vi "BeamCal.vi"() -> ()   [LabVIEW 2022 SP3]
uses:
  -CalTransducer/Hydros.ctl
  -CalTransducer/HydrophoneSettings.ctl
  <vilib>/Analysis/baseanly.llb/Mean (DBL).vi
  <vilib>/Utility/file.llb/Write Delimited Spreadsheet (DBL).vi
  <vilib>/Analysis/2dsp.llb/Zero Padder (DBL).vi
  <vilib>/Analysis/NI_AALPro.lvlib
  <vilib>/Analysis/NI_AALBase.lvlib
panel:
  in  "x*y":dbl[](array[numeric])
  in  "Save P profile":bool
  out "+- Pres":dbl[][](graph)
  in  "Save Path":path
  in  "Next File":bool
  in  "Save Time":bool
  in  "Save Spectra":bool
  in  "View Header?":bool
  in  "Pulse Thresh":dbl=0.025
  out "Data Summary":dbl[](array[numeric])
  in  "ExitSendCmd":bool
  in  "Scale Src":u16(ring)=2 items=["Enter Peak Voltage", "Pk from RF Att ", "Pk from Volt pram"]
  in  "booster amp?":bool=TRUE
  out "Power Spectrum":T1(graph)
  out "StopFreq":dbl format="%.2f"
  out "StartFreq":dbl format="%.2f"
  out "Bandwidth (MHz)\n(6 dB)":dbl format="%.2f"
  out "Max Pulse Parameters":T2 {"pos peak pressure (MPa)" format="%.2f"; "focal length (cm)" format="%.2f"; "MI" format="%.2f"; "Ita.3" format="%.2f"; "Temporal Av Intensity \n(Ita mW/cm^2)" format="%.2f"; "Ipa.3" format="%.2f"; "Pulse Av Intensity\n (Ipa W/cm^2)" format="%.2f"; "Pulse Int \nIntegral (PII J/cm^2)" format="%.2e"; "pulse dur (Pd s)" format="%.3e"; "p.3" format="%.2f"; "neg peak pressure (MPa)" format="%.3f"; "derating (.3) factor" format="%.2f"; "prf" format="%.2f"; "Frequency (MHz)" format="%.2f"}
  out "Power (mW)":dbl format="%.2e"
  in  "Save to file":bool
  out "Isata (mW/cm^2)":dbl format="%.2f"
  in  "pk votage scale (V)":dbl=0.2 format="%.3f"
  out "Raw data":dbl[][](graph)
  out "max line":i32=64
  in  "Hydrophone":T3=enum."DEAD PAL #1818"
  out "beamwidth micron\n(6 dB)":dbl format="%.2f"
  out "Ita":dbl[](graph)
  in  "prf":dbl=1000.0 format="%.2f"
  out "window duration (s)":dbl format="%.2e"
  out "Line":dbl[](graph)
  in  "new file path":path
  in  "Cal Freq (MHz)":dbl=1.0 format="%.2f"
  # "Data is normalized to value of negative peak pressure"
  # "1. Open File (click file image for new path).\n2. Enter parameters (colored fields).\n3. Set Yellow and Red cursors to span pulse.\n4. Adjust Pulse Thresh if necessary.\n5. Most inputs are dynamic and will change values.\n6. To save data, select Save to File on and run VI."
  # "***Voltages are inverted for 40 um PAL devices***"
  # "beam cross sectional\npower"
  # "© 2000-2017 WCM"
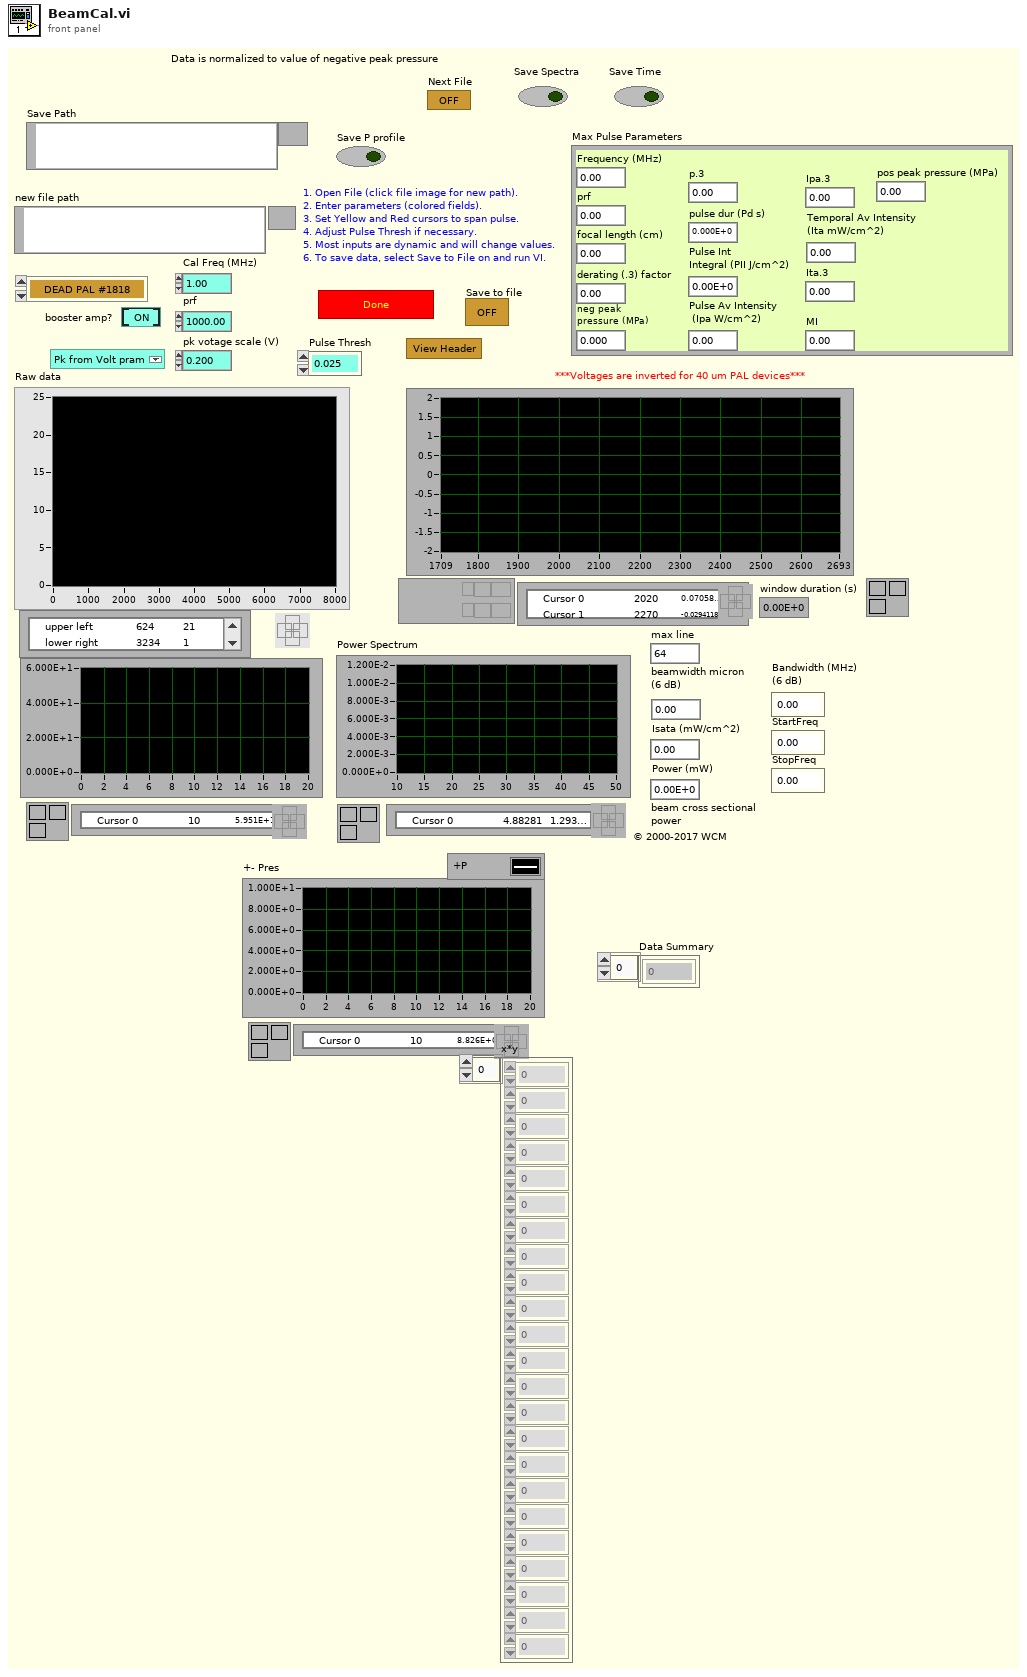
[diagram p1: front panel]
types:
  T1 = cluster{i32, "df":dbl, "Power Spectrum (V^2 rms)":dbl[]}
  T2 = cluster{"Frequency (MHz)":dbl, "prf":dbl, "focal length (cm)":dbl, "derating (.3) factor":dbl, "neg peak pressure (MPa)":dbl, "pos peak pressure (MPa)":dbl, "p.3":dbl, "pulse dur (Pd s)":dbl, "Pulse Int \nIntegral (PII J/cm^2)":dbl, "Pulse Av Intensity\n (Ipa W/cm^2)":dbl, "Ipa.3":dbl, "Temporal Av Intensity \n(Ita mW/cm^2)":dbl, "Ita.3":dbl, "MI":dbl}
  T3 = typedef "Hydros.ctl" = enum16{"PAL #1048", "PAL #525", "PAL #430a", "PAL #192", "DEAD PAL # 1403", "LOST UHI Onda", "DEAD PAL #1818", "PAL #1974", "DEAD #2266 w/booster", "PAL #2524 w/booster", "PAL FP21-20T", "PAL FP160-13  ", "PAL FP141-20", "PAL FP158-08T"}
  T4 = typedef "HydrophoneSettings.ctl" = cluster{"Center Freq (MHz)":dbl, "PRF (kHz)":dbl, "Pulse window (us)":dbl, "Hydrophone":T3, "booster amp?":bool}
  T5 = enum16{"open", "open or create", "create or replace", "create", "open (read only)"}
  T6 = typedef "Header.ctl" = cluster{"header info":cluster{"Header":string, "Head length":i16}, "A/D info":cluster{"# rf points per line":u16, "# lines per scan":u16, "sample rate MHz":u16, "# A/D bits":i16, "# bytes per A/D":u16, "TGC Flag":u16, "A/D Type":string}, "Tranducer Info":cluster{"bandwidth":sgl, "center freq":sgl, "start freq":sgl, "ID":i32}, "Scan Info":cluster{"delay":sgl, "pivot distance":sgl, "sector scan angle":sgl, "operator":string, "Scan Mode":string, "location":string}, "Time/Date Info":cluster{"date":string, "time":string}, "RF Info":cluster{"RF file name":string, "RF file att":string, "RF cal file name":string, "RF cal file att":string}, "Patient Info":cluster{"ID":string, "extended ID":string, "age":u16, "sex":string, "previously\nscanned":string, "PSA":sgl, "LOS":u8, "Ethnicty 2":u8, "Race":u8}, "Tissue Type":cluster{"organ":i16, "disease type":i16, "disease location":i16, "IQ_pts":u16, "RcvBuffer":u8, "RcvFrame":u16, "IQBuff":u8, "IQFrame":u16, "IQPage":u8}, "Votage scaling":cluster{"Digitizer (dB)":sgl, "Gain (dB)":sgl, "Atten (dB)":sgl}, "Comment":string, "Misc Info":cluster{"avg num":u16, "c speed":i16, "Div By or SF zones":i16, "XMIT CHS":u8, "RCV CHS":u8, "Xmit angle":sgl}, "Therapy Parameters":cluster{"Theraputic Freq (MHz)":sgl, "Time on (s)":sgl, "Therapy amplitude (mV)":sgl, "Lines Before":u16, "Lines After":u16}, "Scan Settings":cluster{"Energy (uJ or V)":u8, "Damp (Ohm) or Fc":u8, "HP Filt (KHz)":u8, "LP Filt (MHz)":u8, "Gain (db)":u8, "prf (kHz)":sgl, "Distance between\nscan lines (um)":u16, "Distance between\nscan planes (um)":u16, "Scan line gap (um)":sgl, "Scan plane gap (um)":sgl}, "Compression Parameters":cluster{"F1 (MHz)":sgl, "F2 (MHz)":sgl, "% taper":sgl, "duration":sgl}, "Patient Info Xtra":cluster{"First Name":string, "Last Name":string, "Notes":string}, "ROI Box":u16[]}
  T7 = typedef "LVCursorListTypeDef.ctl" = cluster{"Name":string, "Color":u32, "Style":u8, "Point Style":u8, "Name Visible":bool, "Allow Drag":bool, "Cursor Mode":u32, "Plot":i32, "Index":i32, "Position":cluster{"X":dbl, "Y":dbl}, "X Scale":u32, "Y Scale":u32, "Watch Plots":i32[], "Watch All Plots":bool, "Plot Area":i32, "Label Offset":cluster{"X":dbl, "Y":dbl}}[]
  T8 = cluster{"Name":string, "Color":u32, "Style":u8, "Point Style":u8, "Name Visible":bool, "Allow Drag":bool, "Cursor Mode":u32, "Plot":i32, "Index":i32, "Position":cluster{"X":dbl, "Y":dbl}, "X Scale":u32, "Y Scale":u32, "Watch Plots":i32[], "Watch All Plots":bool, "Plot Area":i32, "Label Offset":cluster{"X":dbl, "Y":dbl}}
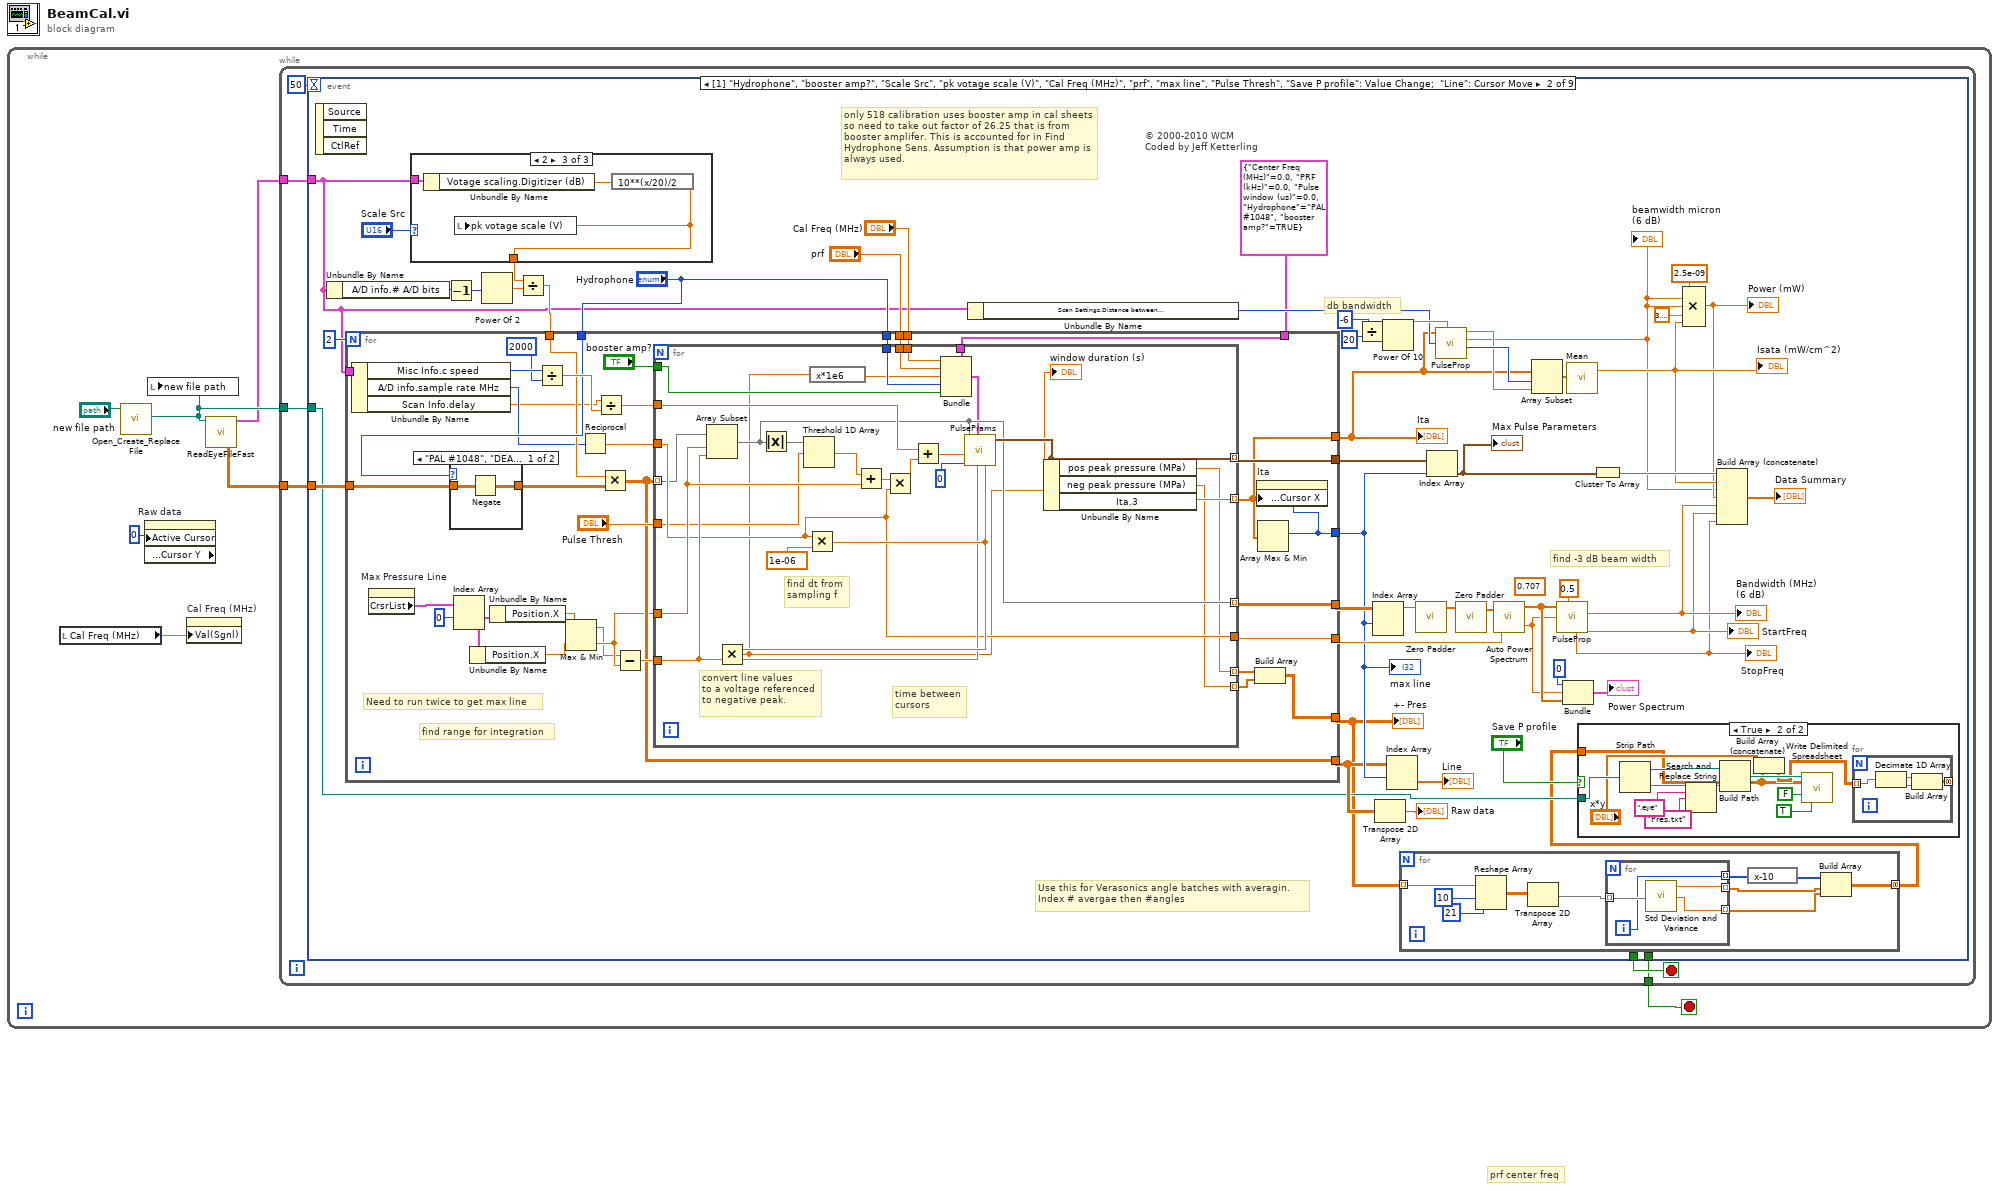
[diagram p0: block diagram]
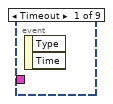
[diagram p2: hidden frame]
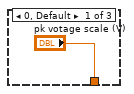
[diagram p5: hidden frame]
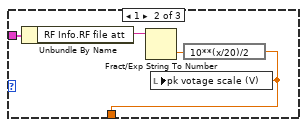
[diagram p6: hidden frame]
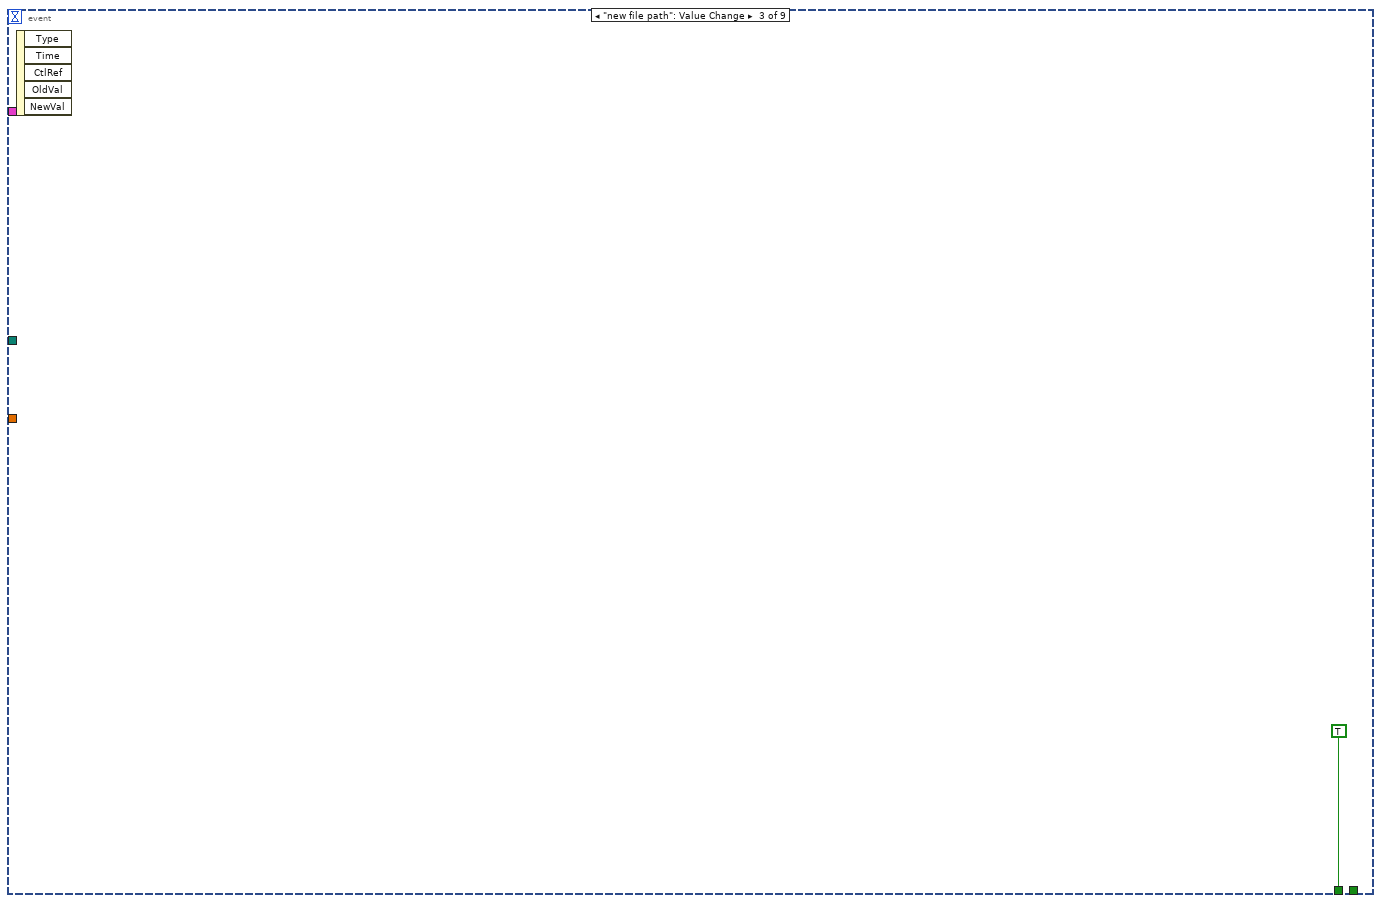
[diagram p7: hidden frame]
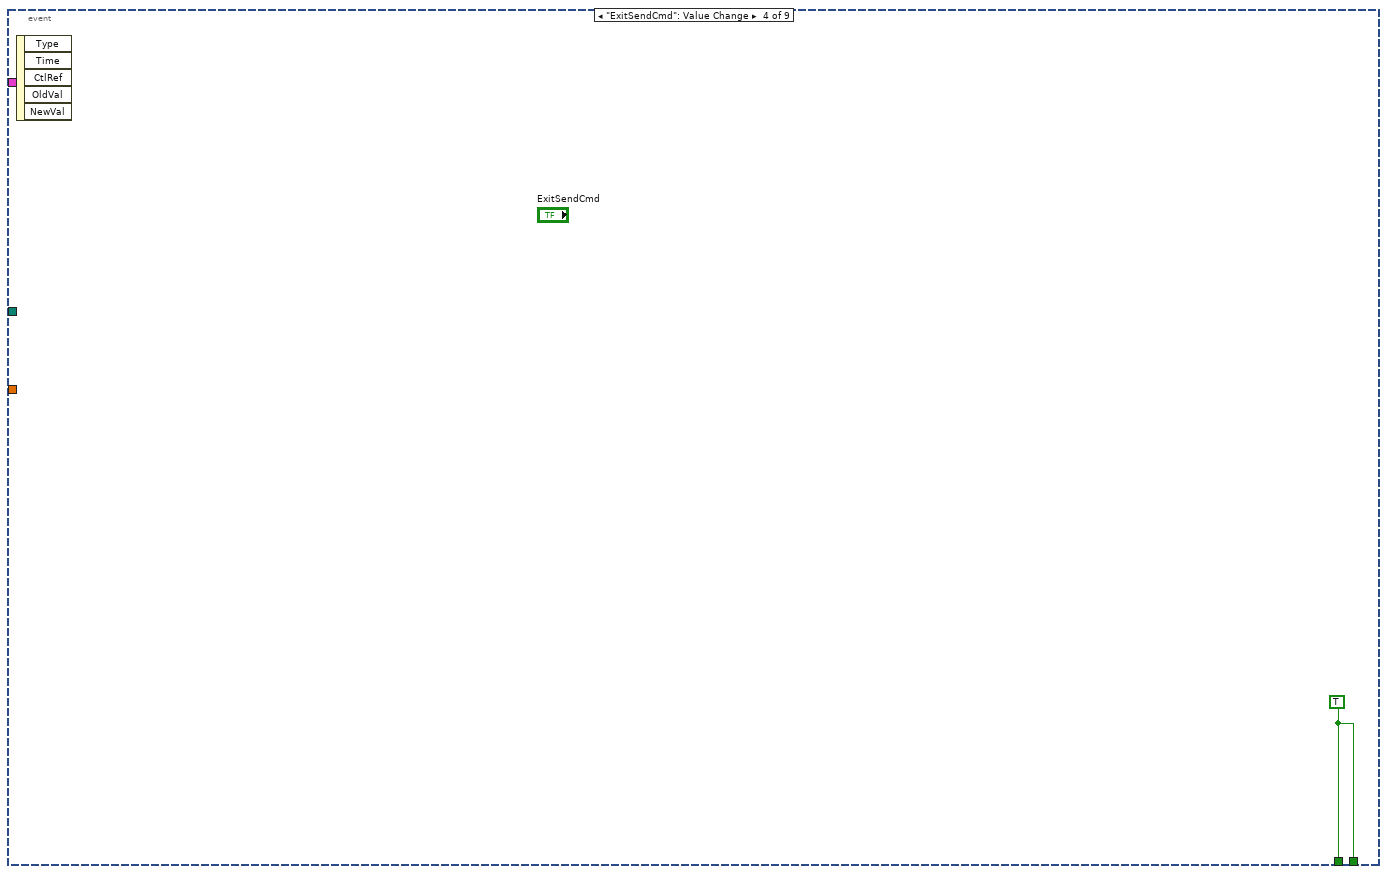
[diagram p8: hidden frame]
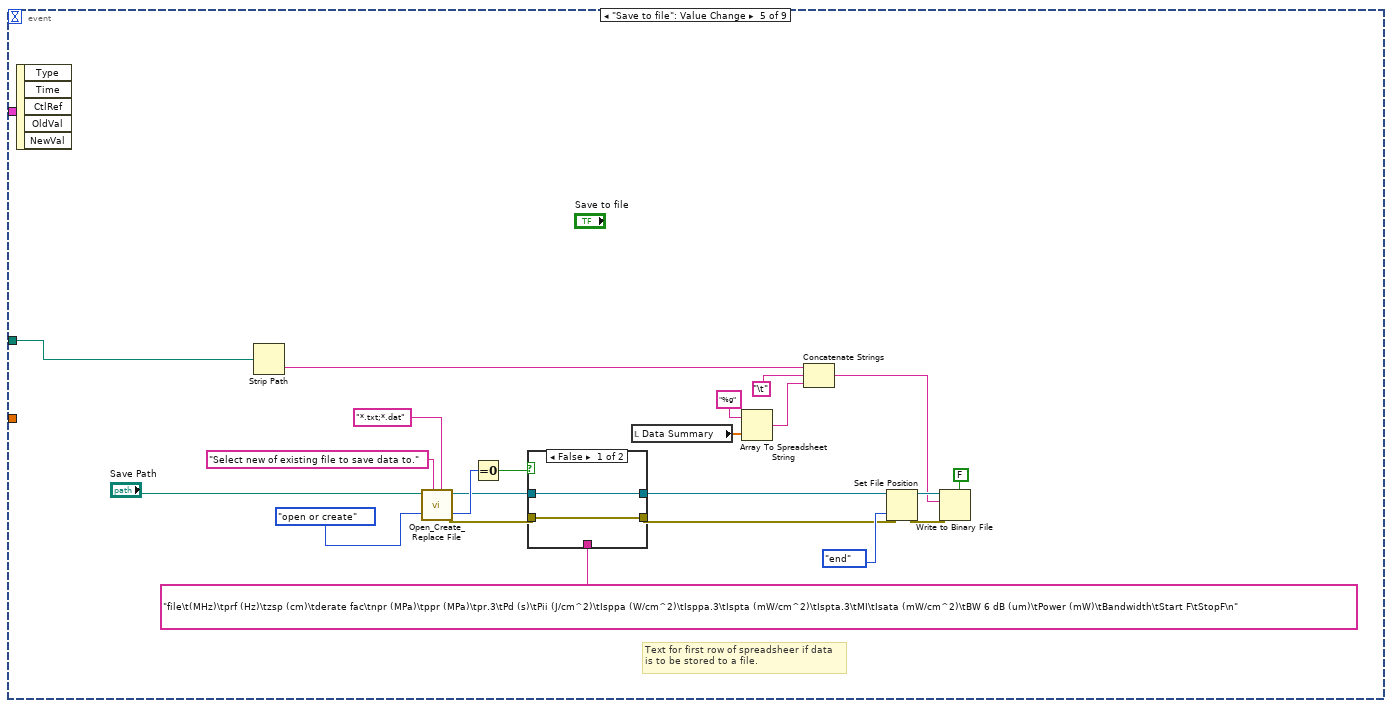
[diagram p9: hidden frame]
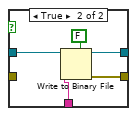
[diagram p10: hidden frame]
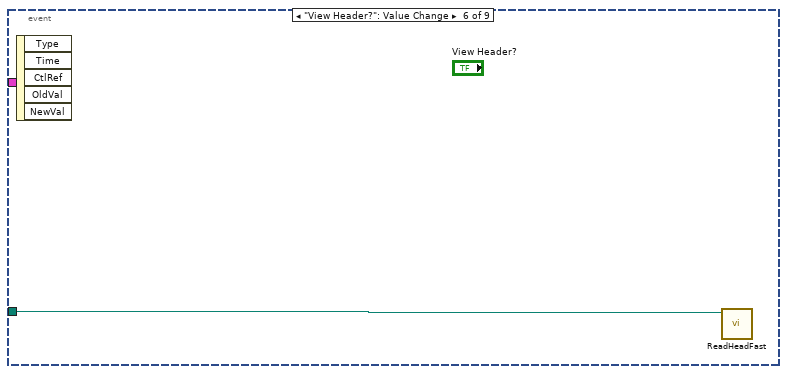
[diagram p11: hidden frame]
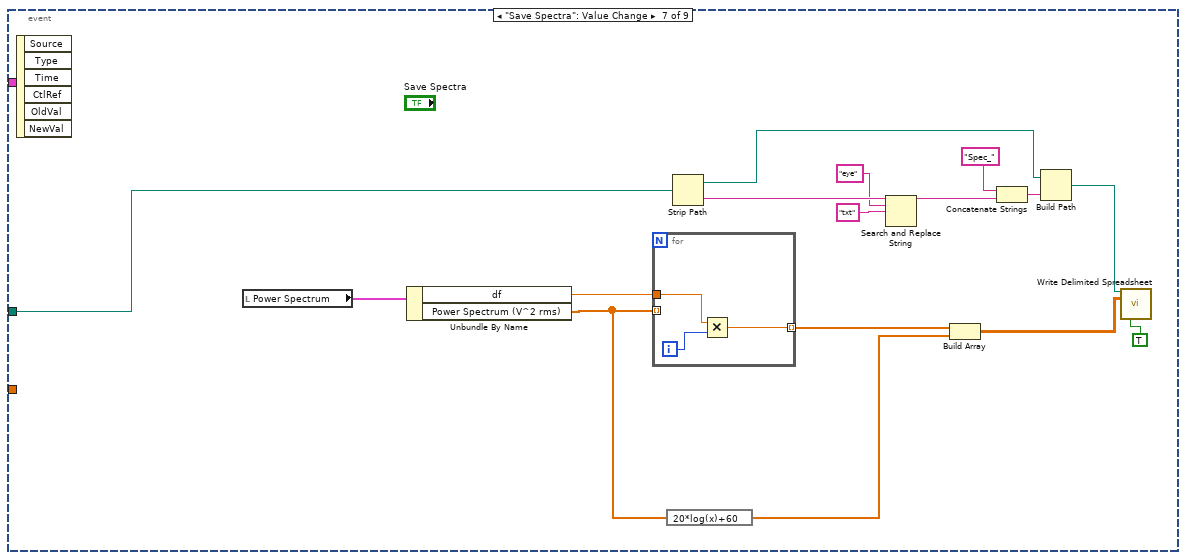
[diagram p12: hidden frame]
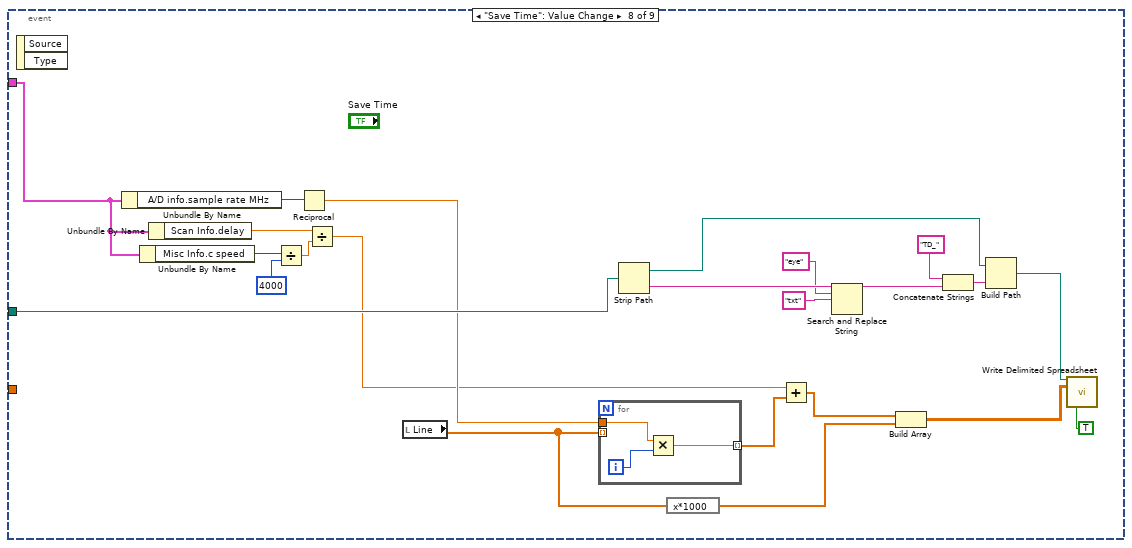
[diagram p13: hidden frame]
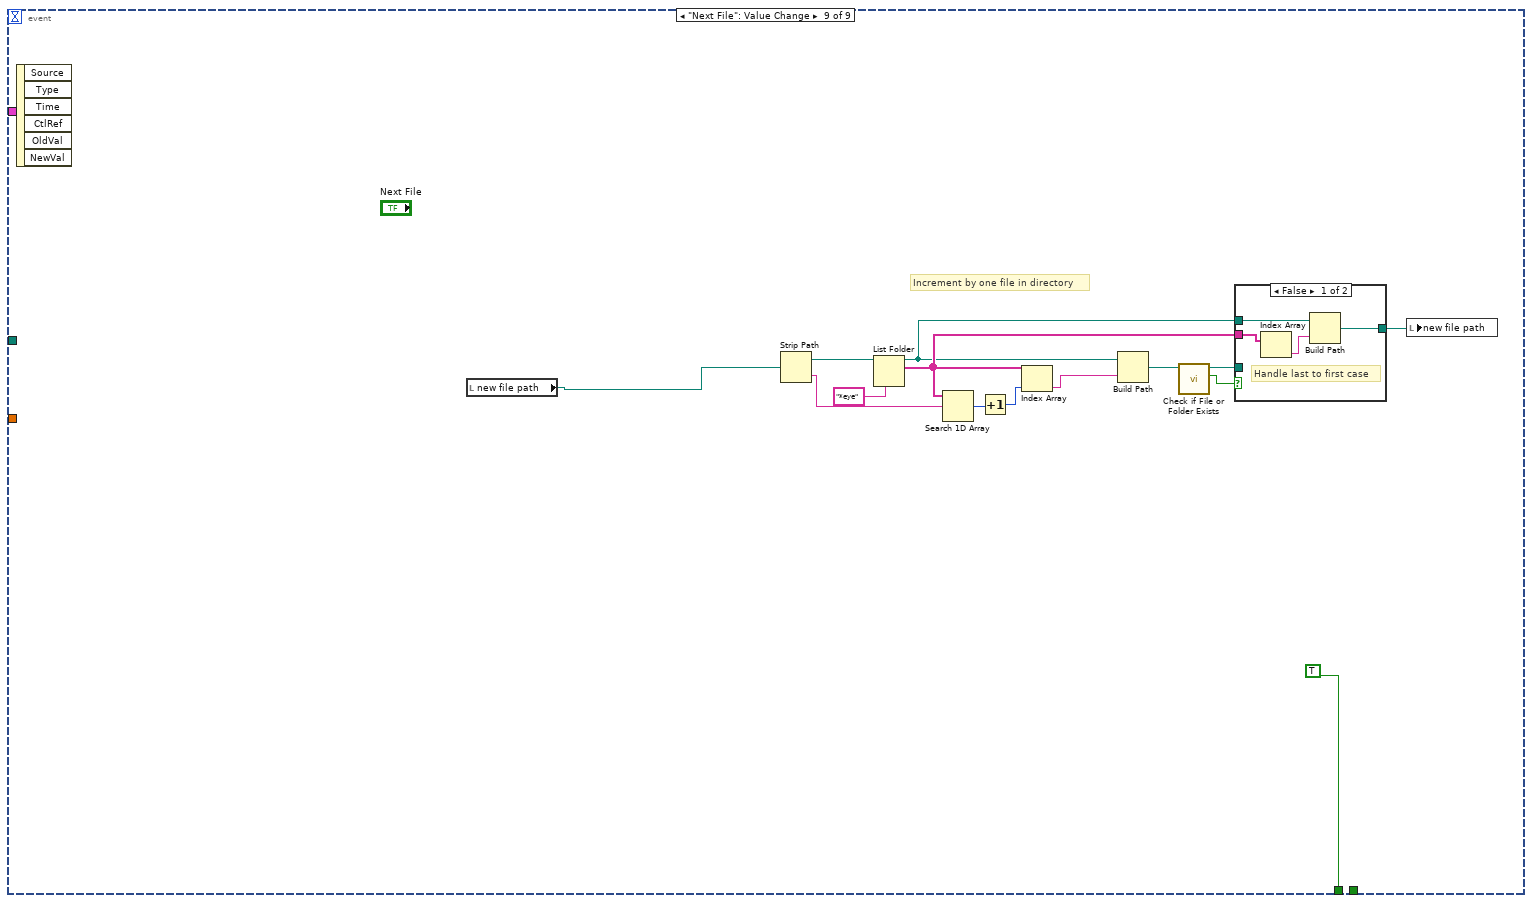
[diagram p14: hidden frame]
diagram:
  # "prf center freq"
  n1 = while {
    stop <- w5 stop-if-true
    n2 = local read "Cal Freq (MHz)"() -> (w4:dbl)
    n3 = call <vilib>:"Open_Create_Replace File.vi"("file path"="new file path") -> ("new file path"=w3:path)  [unwired: 5 in, 5 out]
    n4 = property on="Raw data" class="IntGraph (strict)" props=["Active Cursor", "Cursor", "Cursor Position:Cursor Y"]("Active Cursor"=0) -> ()  [unwired: 2 in, 3 out]
    n5 = local write "new file path"(w3) -> ()
    n6 = property on="Cal Freq (MHz)" class="DigNum (strict)"("Val(Sgnl)"=w4) -> ()  [unwired: 2 in, 2 out]
    n7 = call "ReadEyeFileFast.vi"("new file path"=w3) -> ("2-D data array"=w1:sgl[][], "Header In"=w2:T6)  [unwired: 1 in, 16 out]
    n8 = while {
      tunnel: w1 -> [w13]
      tunnel: [w11] -> w5
      tunnel: w2 -> [w9]
      tunnel: w3 -> [w8]
      stop <- w12 stop-if-true
      n9 = event shown="[1] \"Hydrophone\", \"booster amp?\", \"Scale Src\", \"pk votage scale (V)\", \"Cal Freq (MHz)\", \"prf\", \"max line\", \"Pulse Thresh\", \"Save P profile\": Value Change;  \"Line\": Cursor Move" {
        selector: _ -> [_ _ _ _ _ _ _ _ _]
        dyn-events: _ -> [_ _ _ _ _ _ _ _ _]
        timeout: 50 -> [_ _ _ _ _ _ _ _ _]
        tunnel: w13 -> [_ w32 _ _ _ _ _ _ _]
        tunnel: [_ _ TRUE w171 _ _ _ _ TRUE] -> w12
        tunnel: [_ _ _ w171 _ _ _ _ _] -> w11
        tunnel: w9 -> [_ w20 _ _ _ _ _ w221 _]
        tunnel: w8 -> [_ w16 _ _ w192 w201 w214 w233 _]
        event Timeout {
          n10 = event-data() -> ()  [unwired: 1 in, 2 out]
        }
        event "booster amp?", "Scale Src", "pk votage scale (V)", "Cal Freq (MHz)", "prf", "max line", "Pulse Thresh", "Save P profile": Value Change; "Line": Cursor Move {
          (unwired) 0.707
          # "Use this for Verasonics angle batches with averagin.\nIndex # avergae then #angles"
          # "find -3 dB beam width"
          # "only 518 calibration uses booster amp in cal sheets so need to take out factor of 26.25 that is from booster amplifer. This is accounted for in Find Hydrophone Sens. Assumption is that power amp is always used."
          # "© 2000-2010 WCM\nCoded by Jeff Ketterling"
          # "db bandwidth"
          n11 = event-data() -> ()  [unwired: 1 in, 3 out]
          n12 = Unbundle By Name(w20) -> ("A/D info.# A/D bits"=w29:i16)
          n13 = case shown="2" "Scale Src" {
            tunnel: ["pk votage scale (V)" w163 w169] -> w34
            tunnel: w20 -> [_ w166 w167]
            frame 0, Default {
            }
            frame 1 {
              n14 = Unbundle By Name(w166) -> ("RF Info.RF file att"=w165:string)
              n15 = Fract/Exp String To Number(string=w165) -> (number=w164:dbl)  [unwired: 4 out]
              n16 = expression code="10**(x/20)/2"(w164) -> (w163:dbl)
              n17 = local write "pk votage scale (V)"(w163) -> ()
            }
            frame 2 {
              n18 = Unbundle By Name(w167) -> ("Votage scaling.Digitizer (dB)"=w168:sgl)
              n19 = expression code="10**(x/20)/2"(w168) -> (w169:sgl)
              n20 = local write "pk votage scale (V)"(w169) -> ()
            }
          }
          n21 = Decrement(x=w29) -> (x-1=w28:i16)
          n22 = Power Of 2(x=w28) -> (2^x=w30:dbl)
          n23 = Divide(x=w34, y=w30) -> (x/y=w31:dbl)
          n24 = for {
            N: 2 -> [_]
            tunnel: [w128] -> w18
            tunnel: [w127] -> w57
            tunnel: [w126] -> w55
            tunnel: [w125] -> w22
            tunnel: "Cal Freq (MHz)" -> [w124]
            tunnel: "prf" -> [w123]
            tunnel: "Hydrophone" -> [w122]
            tunnel: w32 -> [w106]
            tunnel: w31 -> [w108]
            tunnel: w20 -> [w114]
            tunnel: [w111] -> w26
            tunnel: [w112] -> w24
            tunnel: "Hydrophone" -> [w110]
            tunnel: T4 {"Center Freq (MHz)"=0.0, "PRF (kHz)"=0.0, "Pulse window (us)"=0.0, "Hydrophone"=enum."PAL #1048", "booster amp?"=TRUE} ("Pressure Cal Parameters") -> [w109]
            tunnel: [w102] -> w15
            # "Need to run twice to get max line"
            # "find range for integration"
            n25 = Unbundle By Name(w114) -> ("Misc Info.c speed"=w118:i16, "A/D info.sample rate MHz"=w105:u16, "Scan Info.delay"=w104:sgl)
            n26 = property on="Max Pressure Line" class="WFGraph (strict)"() -> ("CrsrList"=w130:T7)  [unwired: 2 in, 2 out]
            n27 = case shown="\"PAL #1048\", \"DEAD PAL # 1403\", \"PAL #1974\", \"PAL #2524 w/booster\"" w110 {
              tunnel: w106 -> [w133 w134]
              tunnel: [w132 w134] -> w107
              frame "PAL #1048", "DEAD PAL # 1403", "PAL #1974", "PAL #2524 w/booster" {
                n28 = Negate(x=w133) -> (-x=w132:sgl[][])
              }
              frame "LOST UHI Onda", Default {
              }
            }
            n29 = Index Array(array=w130, index #1=0 ("Index")) -> (element #1=w115:T8, element #2=w96:T8)  [unwired: 1 in]
            n30 = Unbundle By Name(w96) -> ("Position.X"=w99:dbl)
            n31 = Unbundle By Name(w115) -> ("Position.X"=w100:dbl)
            n32 = Divide(x=w118, y=i16 2000) -> (x/y=w116:dbl)
            n33 = Max & Min(x=w100, y=w99) -> (max(x,y)=w97:dbl, min(x,y)=w98:dbl)
            n34 = Reciprocal(x=w105) -> (1/x=w120:dbl)
            n35 = Divide(x=w104, y=w116) -> (x/y=w119:dbl)
            n36 = Multiply(x=w108, y=w107) -> (x*y=w112:dbl[][])
            n37 = Subtract(x=w97, y=w98) -> (x-y=w129:dbl)
            n38 = for {
              tunnel: w98 -> [w158]
              tunnel: w129 -> [w150]
              tunnel: [w151] -> w128 mode=indexing
              tunnel: w120 -> [w147]
              tunnel: w112 -> [w144] mode=indexing
              tunnel: [w160] -> w125 mode=indexing
              tunnel: [w147] -> w127
              tunnel: [w143] -> w126 mode=indexing
              tunnel: w122 -> [w154]
              tunnel: w124 -> [w153]
              tunnel: w123 -> [w152]
              tunnel: "booster amp?" -> [w140]
              tunnel: w119 -> [w148]
              tunnel: "Pulse Thresh" -> [w142]
              tunnel: w109 -> [w139]
              tunnel: [w136] -> w103 mode=indexing
              tunnel: [w135] -> w101 mode=indexing
              # "convert line values\nto a voltage referenced\nto negative peak."
              # "time between\ncursors"
              # "find dt from\nsampling f"
              n39 = Array Subset(array=w144, index=w158, length=w150) -> (w143:dbl[])
              n40 = Absolute Value(x=w143) -> (abs(x)=w146:dbl[])
              n41 = Threshold 1D Array(2:w142, 3:w146) -> (0:w145:dbl)  [unwired: 1 out]
              n42 = Multiply(x=w147, y=1e-06 ("x")) -> (x*y=w156:dbl)
              n43 = Multiply(x=w156, y=w150) -> (x*y=w138:dbl)
              "window duration (s)" <- w138
              n44 = expression code="x*1e6"(w138) -> (w137:dbl)
              n45 = Add(x=w145, y=w158) -> (x+y=w157:dbl)
              n46 = Multiply(x=w157, y=w147) -> (x*y=w159:dbl)
              n47 = Add(x=w148, y=w159) -> (x+y=w155:dbl)
              n48 = Bundle(cluster=w139, "Center Freq (MHz)"=w153, "PRF (kHz)"=w152, "Pulse window (us)"=w137, "Hydrophone"=w154, "booster amp?"=w140) -> (w141:T4)
              n49 = call "PulsePrams.vi"("sample rate (s/Pt)"=w156, "Length of Subset"=w150, "Pressure Cal Parameters"=w141, "Index of subset"=0, "delay (ms)"=w155, "Data"=w143) -> ("Pulse Parameters"=w151:T2)  [unwired: 1 in, 4 out]
              n50 = Unbundle By Name(w151) -> ("pos peak pressure (MPa)"=w136:dbl, "neg peak pressure (MPa)"=w135:dbl, "Ita.3"=w160:dbl)
            }
            n51 = Build Array(w103, w101) -> (w102:dbl[][])
            n52 = Array Max & Min(array=w125) -> (max index (indices)=w111:i32)  [unwired: 3 out]
            n53 = property on="Ita" class="WFGraph (strict)"("Cursor.Cursor Position:Cursor X"=w111) -> ()  [unwired: 2 in, 2 out]
          }
          "Ita" <- w22
          "max line" <- w26
          "+- Pres" <- w15
          n54 = Unbundle By Name(w20) -> ("Scan Settings.Distance between\nscan lines (um)"=w40:u16)
          n55 = Divide(x=-6, y=20) -> (x/y=w63:dbl)
          n56 = Index Array(array=w55, index (row)=w26) -> (element=w54:dbl[])  [unwired: 1 in]
          n57 = Transpose 2D Array(2D array=w24) -> (transposed array=→"Raw data":dbl[][])
          n58 = Power Of 10(x=w63) -> (10^x=w56:dbl)
          n59 = Index Array(array=w24, index (row)=w26) -> (element=→"Line":dbl[])  [unwired: 1 in]
          n60 = for {
            tunnel: w15 -> [w75] mode=indexing
            tunnel: [w66] -> w14 mode=concatenating
            n61 = Reshape Array(w75, 10 ("dimension size"), 21 ("dimension size")) -> (w72:dbl[][])
            n62 = Transpose 2D Array(2D array=w72) -> (transposed array=w67:dbl[][])
            n63 = for {
              tunnel: w67 -> [w79] mode=indexing
              tunnel: [w78] -> w69 mode=indexing
              tunnel: [w77] -> w68 mode=indexing
              tunnel: [w76] -> w71 mode=indexing
              i -> [w76]
              n64 = call <vilib>:"Std Deviation and Variance.vi"("X"=w79) -> ("mean"=w78:dbl, "standard deviation"=w77:dbl)  [unwired: 1 in, 1 out]
            }
            n65 = expression code="x-10"(w71) -> (w70:i32[])
            n66 = Build Array(w70, w69, w68) -> (w66:dbl[][])
          }
          n67 = call-poly <vilib>:"Zero Padder.vi"("Input Array"=w54) -> ("Zero Padded Array"=w49:dbl[])  [unwired: 1 in, 9 out]
          n68 = Index Array(array=w18, index=w26) -> (element=w58:T2)
          "Max Pulse Parameters" <- w58
          n69 = call "PulseProp.vi"("Data"=w22, "Scale factor"=w56, "spacing"=w40) -> ("Pts in range"=w47:dbl, "width"=w44:dbl, "Start pt"=w48:i32)  [unwired: 1 in, 4 out]
          "beamwidth micron\n(6 dB)" <- w44
          n70 = call-poly <vilib>:"Zero Padder.vi"("Input Array"=w49) -> ("Zero Padded Array"=w53:dbl[])  [unwired: 1 in, 9 out]
          n71 = call <vilib>:"Auto Power Spectrum.vi"("dt"=w57, "Signal (V)"=w53) -> ("df"=w36:dbl, "Power Spectrum (V^2 rms)"=w38:dbl[])
          n72 = Array Subset(array=w22, index=w48, length=w47) -> (w61:dbl[])
          n73 = call "PulseProp.vi"("Data"=w38, "Scale factor"=0.5, "spacing"=w36) -> ("width"=w52:dbl, "StopValue"=w50:dbl, "StartValue"=w51:dbl)  [unwired: 2 in, 3 out]
          "Bandwidth (MHz)\n(6 dB)" <- w52
          "StartFreq" <- w51
          "StopFreq" <- w50
          n74 = Bundle(0, "df"=w36, "Power Spectrum (V^2 rms)"=w38) -> (→"Power Spectrum":T1)  [unwired: 1 out]
          n75 = call-poly <vilib>:"Mean.vi"("X"=w61) -> ("mean"=w59:dbl)  [unwired: 1 out]
          "Isata (mW/cm^2)" <- w59
          n76 = case shown="True" "Save P profile" {
            tunnel: w14 -> [_ w80]
            tunnel: w16 -> [_ w83]
            frame False {
            }
            frame True {
              n77 = Strip Path(path=w83) -> (stripped path=w86:path, name=w89:string)
              n78 = Search and Replace String(input string=w89, search string=".eye", replace string="Pres.txt" ("replace string (\"\")")) -> (result string=w85:string)  [unwired: 5 in, 3 out]
              n79 = Build Path(base path=w86, name or relative path=w85) -> (appended path=w84:path)
              n80 = Build Array (concatenate)("x*y", w80) -> (w81:dbl[][])
              n81 = call-poly <vilib>:"Write Delimited Spreadsheet.vi"("file path (dialog if empty)"=w84, "2D data"=w80, "append to file? (new file:F)"=FALSE, "transpose? (no:F)"=TRUE) -> ()  [unwired: 10 in, 2 out]
              n82 = for {
                tunnel: w81 -> [w95] mode=indexing
                tunnel: [w92] -> _ mode=concatenating
                n83 = Decimate 1D Array(w95) -> (w93:dbl[], w94:dbl[])
                n84 = Build Array(w93, w94) -> (w92:dbl[][])
              }
            }
          }
          n85 = Cluster To Array(cluster=w58) -> (array=w62:dbl[])
          n86 = Compound Arithmetic op=MULTIPLY(2.5e-09, w44, w44, 3.141592653589793, w59) -> (w46:dbl)
          "Power (mW)" <- w46
          n87 = Build Array (concatenate)(w62, w59, w44, w46, w52, w51, w50) -> (→"Data Summary":dbl[])
        }
        event "new file path": Value Change {
          n88 = event-data() -> ()  [unwired: 1 in, 5 out]
        }
        event "ExitSendCmd": Value Change {
          w171 = TRUE
          n89 = event-data() -> ()  [unwired: 1 in, 5 out]
        }
        event "Save to file": Value Change {
          # "Text for first row of spreadsheer if data\nis to be stored to a file."
          n90 = event-data() -> ()  [unwired: 1 in, 5 out]
          n91 = Strip Path(path=w192) -> (name=w179:string)  [unwired: 1 out]
          n92 = call <vilib>:"Open_Create_Replace File.vi"("pattern"="*.txt;*.dat", "prompt"="Select new of existing file to save data to.", "function (open:0)"=T5."open or create", "file path"="Save Path") -> ("error out"=w174:errorcluster, "file size (bytes)"=w183:i32, "refnum"=w180:refnum<file>)  [unwired: 3 in, 2 out]
          n93 = Equal To 0?(x=w183) -> (x = 0?=w182:bool)
          n94 = case shown="False" w182 {
            tunnel: "file\t(MHz)\tprf (Hz)\tzsp (cm)\tderate fac\tnpr (MPa)\tppr (MPa)\tpr.3\tPd (s)\tPii (J/cm^2)\tIsppa (W/cm^2)\tIsppa.3\tIspta (mW/cm^2)\tIspta.3\tMI\tIsata (mW/cm^2)\tBW 6 dB (um)\tPower (mW)\tBandwidth\tStart F\tStopF\n" -> [_ w198]
            tunnel: [w195 w199] -> w178
            tunnel: w180 -> [w195 w200]
            tunnel: [w194 w196] -> w175
            tunnel: w174 -> [w194 _]
            frame False {
            }
            frame True {
              n95 = Write to Binary File(file (use dialog)=w200, data=w198, 5:FALSE ("prepend array or string size? (T)")) -> (refnum out=w199:refnum<file>, error out=w196:errorcluster)  [unwired: 1 in, 3 out]
            }
          }
          n96 = local read "Data Summary"() -> (w176:dbl[])
          n97 = Array To Spreadsheet String(array=w176, 3:"%g" ("format string")) -> (spreadsheet string=w186:string)  [unwired: 1 out]
          n98 = Concatenate Strings(w179, "\t", w186) -> (w188:string)
          n99 = Set File Position(refnum=w178, from (0:start)=enum16{"start", "end", "current"}."end" ("pos mode (0:2)"), error in=w175) -> (refnum out=w190:refnum<file>, error out=w191:errorcluster)  [unwired: 1 out]
          n100 = Write to Binary File(file (use dialog)=w190, data=w188, error in=w191, 5:FALSE ("prepend array or string size? (T)")) -> ()  [unwired: 5 out]
        }
        event "View Header?": Value Change {
          n101 = event-data() -> ()  [unwired: 1 in, 5 out]
          n102 = call "ReadHeadFast.vi"("new file path"=w201) -> ()  [unwired: 7 in, 4 out]
        }
        event "Save Spectra": Value Change {
          n103 = event-data() -> ()  [unwired: 1 in, 6 out]
          n104 = local read "Power Spectrum"() -> (w217:T1)
          n105 = Unbundle By Name(w217) -> ("df"=w216:dbl, "Power Spectrum (V^2 rms)"=w203:dbl[])
          n106 = for {
            tunnel: w203 -> [_] mode=indexing
            tunnel: w216 -> [w219]
            tunnel: [w218] -> w215 mode=indexing
            i -> [w220]
            n107 = Multiply(x=w219, y=w220) -> (x*y=w218:dbl)
          }
          n108 = expression code="20*log(x)+60"(w203) -> (w202:dbl[])
          n109 = Strip Path(path=w214) -> (stripped path=w207:path, name=w213:string)
          n110 = Search and Replace String(input string=w213, search string="eye", replace string="txt" ("replace string (\"\")")) -> (result string=w210:string)  [unwired: 5 in, 3 out]
          n111 = Build Array(w215, w202) -> (w205:dbl[][])
          n112 = Concatenate Strings("Spec_" ("string"), w210) -> (w208:string)
          n113 = Build Path(base path=w207, name or relative path=w208) -> (appended path=w206:path)
          n114 = call-poly <vilib>:"Write Delimited Spreadsheet.vi"("file path (dialog if empty)"=w206, "2D data"=w205, "transpose? (no:F)"=TRUE) -> ()  [unwired: 11 in, 2 out]
        }
        event "Save Time": Value Change {
          n115 = event-data() -> ()  [unwired: 1 in, 2 out]
          n116 = Unbundle By Name(w221) -> ("A/D info.sample rate MHz"=w232:u16)
          n117 = Unbundle By Name(w221) -> ("Misc Info.c speed"=w229:i16)
          n118 = Unbundle By Name(w221) -> ("Scan Info.delay"=w230:sgl)
          n119 = Divide(x=w229, y=i16 4000) -> (x/y=w228:dbl)
          n120 = Reciprocal(x=w232) -> (1/x=w231:dbl)
          n121 = Divide(x=w230, y=w228) -> (x/y=w225:dbl)
          n122 = local read "Line"() -> (w223:dbl[])
          n123 = for {
            tunnel: w223 -> [_] mode=indexing
            tunnel: w231 -> [w245]
            tunnel: [w244] -> w226 mode=indexing
            i -> [w246]
            n124 = Multiply(x=w245, y=w246) -> (x*y=w244:dbl)
          }
          n125 = Strip Path(path=w233) -> (stripped path=w237:path, name=w243:string)
          n126 = expression code="x*1000"(w223) -> (w222:dbl[])
          n127 = Add(x=w225, y=w226) -> (x+y=w224:dbl[])
          n128 = Search and Replace String(input string=w243, search string="eye", replace string="txt" ("replace string (\"\")")) -> (result string=w240:string)  [unwired: 5 in, 3 out]
          n129 = Build Array(w224, w222) -> (w235:dbl[][])
          n130 = Concatenate Strings("TD_" ("string"), w240) -> (w238:string)
          n131 = Build Path(base path=w237, name or relative path=w238) -> (appended path=w236:path)
          n132 = call-poly <vilib>:"Write Delimited Spreadsheet.vi"("file path (dialog if empty)"=w236, "2D data"=w235, "transpose? (no:F)"=TRUE) -> ()  [unwired: 11 in, 2 out]
        }
        event "Next File": Value Change {
          # "Increment by one file in directory"
          n133 = event-data() -> ()  [unwired: 1 in, 6 out]
          n134 = local read "new file path"() -> (w250:path)
          n135 = Strip Path(path=w250) -> (stripped path=w252:path, name=w260:string)
          n136 = List Folder(path=w252, pattern="*eye") -> (path out=w253:path, filenames=w254:string[])  [unwired: 1 in, 3 out]
          n137 = Search 1D Array(1D array=w254, element=w260) -> (index of element=w259:i32)  [unwired: 1 out]
          n138 = Increment(x=w259) -> (x+1=w258:i32)
          n139 = Index Array(array=w254, index=w258) -> (element=w257:string)
          n140 = Build Path(base path=w253, name or relative path=w257) -> (appended path=w251:path)
          n141 = call <vilib>:"Check if File or Folder Exists.vi"("path"=w251) -> ("file or folder exists?"=w255:bool, "dup path"=w256:path)  [unwired: 1 in, 8 out]
          n142 = case shown="False" w255 {
            tunnel: w256 -> [_ w265]
            tunnel: w254 -> [w264 _]
            tunnel: w253 -> [w263 _]
            tunnel: [w261 w265] -> w249
            frame False {
              # "Handle last to first case"
              n143 = Index Array(array=w264) -> (element=w262:string)  [unwired: 1 in]
              n144 = Build Path(base path=w263, name or relative path=w262) -> (appended path=w261:path)
            }
            frame True {
            }
          }
          n145 = local write "new file path"(w249) -> ()
        }
      }
    }
  }
